vi "Green Channel.vi"(2 "Error":string, 3 "Image":T1={"Image ID"=0, "Channel ID"=-1}) -> (0 "Error":string, 1 "Image":T1={"Image ID"=0, "Channel ID"=-1})   [LabVIEW 2011, in "labvvis.lvlib"]
doc: "Provides access to the Green channel in a RGBA image. Modifying the resultant \"image\" will actually modify the channel in the original image."
uses:
  <userlib>/labvvis/labvvis.lvlib
  <userlib>/labvvis/VVIS Image.ctl
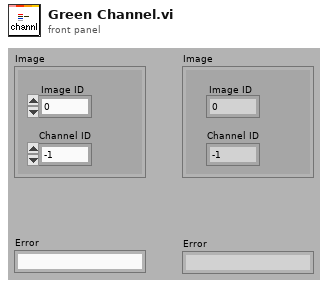
[diagram p1: front panel]
types:
  T1 = typedef "labvvis.lvlib/VVIS Image.ctl" = cluster{"Image ID":i16, "Channel ID":i16}
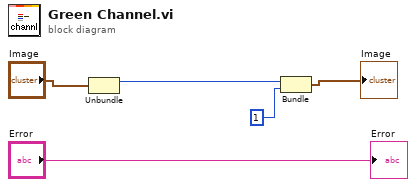
[diagram p0: block diagram]
diagram:
  n1 = Unbundle("Image") -> ("Image ID"=w5:i16)  [unwired: 1 out]
  n2 = Bundle("Image ID"=w5, i16 1) -> (→"Image":cluster{"Image ID":i16, i16})  [unwired: 1 in]
  "Error" <- "Error"
